vi "M_alpha_beta_2 (SubVI).vi"(4 "i":i32, 7 "FE [N]":dbl[](array[numeric]), 8 "Vehicle Parameters":T1, 10 "Data":dbl[][](array[numeric]), 11 "cluster":T3) -> (0 "output cluster":T2, 2 "M_beta":dbl, 3 "M_alpha":dbl)   [LabVIEW 2017]
uses:
  <vilib>/Analysis/_algsub.llb/Vector Norm Type.ctl
  <vilib>/Analysis/_algsub.llb/Real Vector Norm.vi
  <vilib>/Analysis/NI_AALPro.lvlib
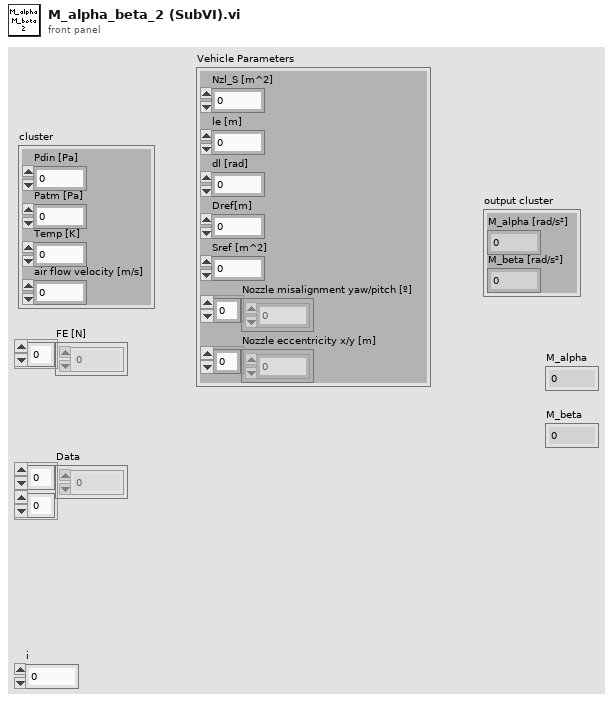
[diagram p1: front panel]
types:
  T1 = cluster{"Nzl_S [m^2]":dbl, "le [m]":dbl, "dl [rad]":dbl, "Dref[m]":dbl, "Sref [m^2]":dbl, "Nozzle misalignment yaw/pitch [º]":dbl[], "Nozzle eccentricity x/y [m]":dbl[]}
  T2 = cluster{"M_alpha [rad/s²]":dbl, "M_beta [rad/s²]":dbl}
  T3 = cluster{"Pdin [Pa]":dbl, "Patm [Pa]":dbl, "Temp [K]":dbl, "air flow velocity [m/s]":dbl}
  T4 = typedef "NI_AALPro.lvlib/Vector Norm Type.ctl" = u16
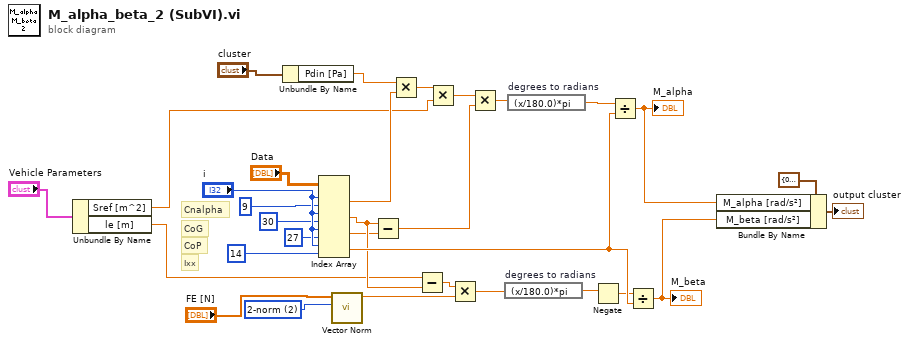
[diagram p0: block diagram]
diagram:
  w24 = T4 2 items=["1-norm"=1, "2-norm"=2, "Inf-norm"=3, "-Inf-norm"=4, "User Defined"=5] ("norm type")
  # "Ixx"
  # "CoP"
  # "CoG"
  # "Cnalpha"
  n1 = Unbundle By Name("Vehicle Parameters") -> ("Sref [m^2]"=w6:dbl, "le [m]"=w7:dbl)
  n2 = Unbundle By Name("cluster") -> ("Pdin [Pa]"=w9:dbl)
  n3 = Index Array(array="Data", index (row) #1="i", index (col) #1=9 ("disabled index (col)"), index (row) #2="i", index (col) #2=30 ("disabled index (col)"), index (row) #3="i", index (col) #3=27 ("disabled index (col)"), index (row) #4="i", index (col) #4=14 ("disabled index (col)")) -> (element #1=w22:dbl, element #2=w25:dbl, element #3=w17:dbl, element #4=w31:dbl)
  n4 = call-poly <vilib>:"Vector Norm.vi"("norm type"=w24, "Input Vector"="FE [N]") -> ("norm"=w26:dbl)  [unwired: 8 in, 1 out]
  n5 = Subtract(x=w25, y=w17) -> (x-y=w19:dbl)
  n6 = Multiply(x=w9, y=w22) -> (x*y=w16:dbl)
  n7 = Subtract(x=w7, y=w25) -> (x-y=w27:dbl)
  n8 = Multiply(x=w16, y=w6) -> (x*y=w18:dbl)
  n9 = Multiply(x=w27, y=w26) -> (x*y=w28:dbl)
  n10 = Multiply(x=w18, y=w19) -> (x*y=w20:dbl)
  n11 = expression code="(x/180.0)*pi" "degrees to radians"(w28) -> (w29:dbl)
  n12 = expression code="(x/180.0)*pi" "degrees to radians"(w20) -> (w21:dbl)
  n13 = Negate(x=w29) -> (-x=w30:dbl)
  n14 = Divide(x=w21, y=w31) -> (x/y=w4:dbl)
  "M_alpha" <- w4
  n15 = Divide(x=w30, y=w31) -> (x/y=w3:dbl)
  "M_beta" <- w3
  n16 = Bundle By Name(cluster=T2 {"M_alpha [rad/s²]"=0.0, "M_beta [rad/s²]"=0.0} ("output cluster 2"), "M_alpha [rad/s²]"=w4, "M_beta [rad/s²]"=w3) -> (→"output cluster":T2)
